vi "theta0.vi"(4 "L1":i32, 6 "X":i32, 7 "L0":i32, 8 "theta 1":i32, 9 "Y":i32) -> (11 "theta 0":dbl)   [LabVIEW 2014]
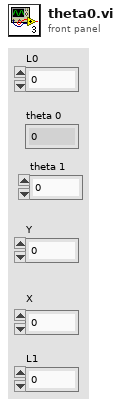
[diagram p1: front panel]
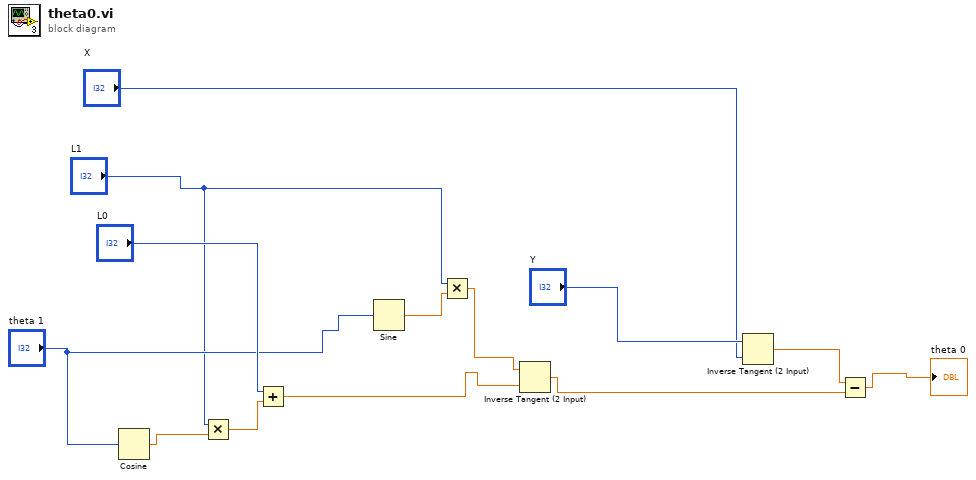
[diagram p0: block diagram]
diagram:
  n1 = Cosine(x="theta 1") -> (cos(x)=w8:dbl)
  n2 = Multiply(x="L1", y=w8) -> (x*y=w6:dbl)
  n3 = Add(x="L0", y=w6) -> (x+y=w3:dbl)
  n4 = Sine(x="theta 1") -> (sin(x)=w5:dbl)
  n5 = Multiply(x="L1", y=w5) -> (x*y=w4:dbl)
  n6 = Inverse Tangent (2 Input)(1:w3, 2:w4) -> (0:w12:dbl)
  n7 = Inverse Tangent (2 Input)(1:"X", 2:"Y") -> (0:w11:dbl)
  n8 = Subtract(x=w11, y=w12) -> (x-y=→"theta 0":dbl)
